vi "Read SerialCommunicator.vi"(8 "error in (no error)":errorcluster, 11 "SerialClient in":refnum<class "SerialCommunication.lvclass">) -> (0 "error out":errorcluster, 2 "SerialProtocols.lvlib:SerialCommunicator.lvclass":refnum<class "SerialCommunicator.lvclass">, 3 "SerialClient out":refnum<class "SerialCommunication.lvclass">)   [LabVIEW 2016, in "SerialCommunication.lvclass"]
uses:
  SerialCommunication.lvclass
  common_serialprotocols/SerialCommunicator/SerialCommunicator.lvclass
  SerialCommunication.lvclass/SerialCommunication.ctl
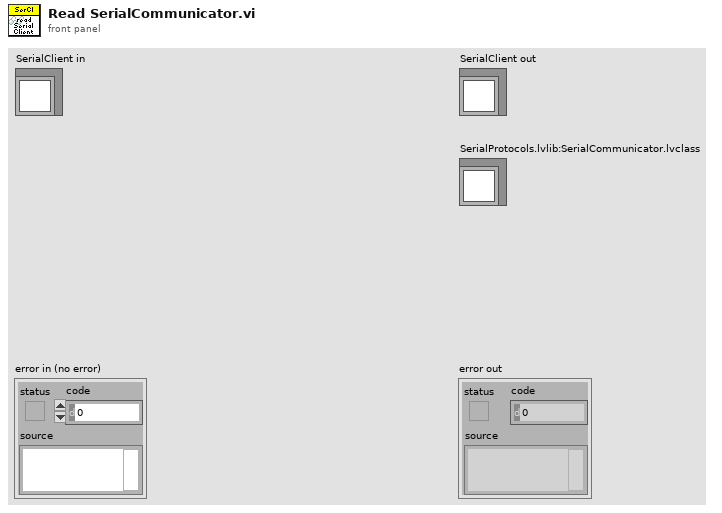
[diagram p1: front panel]
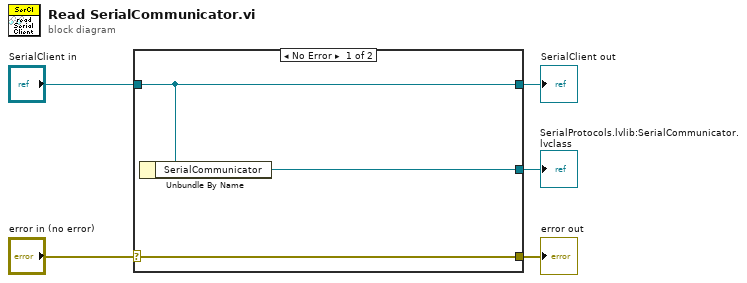
[diagram p0: block diagram]
diagram:
  n1 = case shown="No Error" "error in (no error)" {
    selector: "error in (no error)" -> [w8 w9]
    tunnel: [w8 w9] -> w4
    tunnel: [w7 w10] -> w2
    tunnel: "SerialClient in" -> [w7 w10]
    tunnel: [w6 _] -> w1
    frame No Error {
      n2 = Unbundle By Name(w7) -> ("SerialCommunicator"=w6:refnum<class "SerialCommunicator.lvclass">)
    }
    frame Error {
    }
  }
  "error out" <- w4
  "SerialClient out" <- w2
  "SerialProtocols.lvlib:SerialCommunicator.lvclass" <- w1
